vi "Debug Exercise (Main).vi"() -> ()   [LabVIEW 2019]
doc: "This VI is part of Exercise 2-3 in the LabVIEW Basics I Course.\n\nFirst, fix the broken run arrow and then use the different debugging tools to see how they work."
panel:
  in  "Stop Button":bool
  out "Final Result":dbl format="%.2f"
  out "Random Number":dbl format="%.2f"
  out "Multiply Result":dbl format="%.2f"
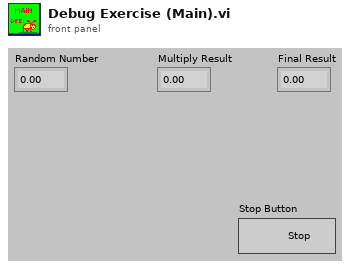
[diagram p1: front panel]
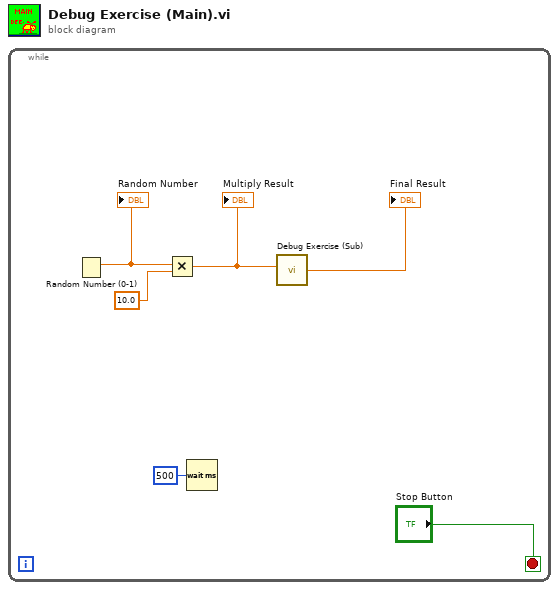
[diagram p0: block diagram]
diagram:
  n1 = while {
    stop <- "Stop Button" stop-if-true
    n2 = Random Number (0-1)() -> (number: 0 to 1=w5:dbl)
    "Random Number" <- w5
    n3 = Multiply(x=w5, y=10.0) -> (x*y=w6:dbl)
    "Multiply Result" <- w6
    n4 = Wait (ms)(milliseconds to wait=u32 500) -> ()  [unwired: 1 out]
    n5 = call "Debug Exercise (Sub).vi"("Number"=w6) -> ("Final Result"=→"Final Result":dbl)
  }
